vi "_AllThingsVIA.vi"   [LabVIEW 2012]
uses:
  <vilib>/NXT/LegoClasses/VIA/VIA.lvclass
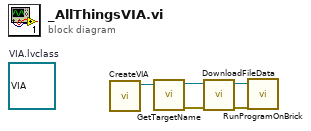
[diagram p0: block diagram]
diagram:
  (unwired) refnum<class "VIA.lvclass"> refnum  # VIA.lvclass
  n1 = call <vilib>:"CreateVIA.vi"() -> ("VIA.lvclass"=w5:refnum<class "VIA.lvclass">)  [unwired: 11 in]
  n2 = call-dynamic "GetTargetName.vi"("VIA in"=w5) -> ("error out"=w4:errorcluster, "VIA out"=w3:refnum<class "VIA.lvclass">)  [unwired: 8 in, 1 out]
  n3 = call-dynamic "DownloadFileData.vi"("error in (no error)"=w4, "VIA in"=w3) -> ("error out"=w2:errorcluster, "VIA out"=w1:refnum<class "VIA.lvclass">)  [unwired: 6 in, 2 out]
  n4 = call-dynamic "RunProgramOnBrick.vi"("error in (no error)"=w2, "VIA in"=w1) -> ()  [unwired: 8 in, 2 out]
